vi "SM_S700_Serial_String_Identify.vi"(11 "read buffer":string) -> (3 "selection":bool)   [LabVIEW 2011]
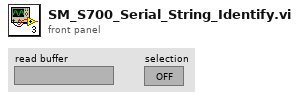
[diagram p1: front panel]
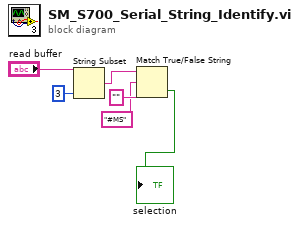
[diagram p0: block diagram]
diagram:
  n1 = String Subset(string="read buffer", length (rest)=3 ("length (rest)")) -> (substring=w2:string)  [unwired: 1 in]
  n2 = Match True/False String(2:"" ("false string"), 3:"#MS" ("true string"), 4:w2) -> (0:→"selection":bool)  [unwired: 1 out]
